vi "Untitled 3.vi"() -> ()   [LabVIEW 2017]
uses:
  8dd77c05-3ed4-427d-9456-dd24b11b0c44.vi
panel:
  out "<JSON>":string
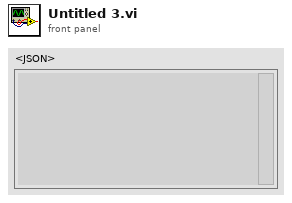
[diagram p1: front panel]
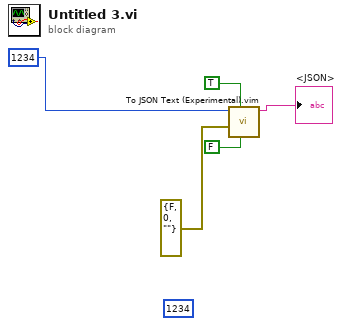
[diagram p0: block diagram]
diagram:
  (unwired) 1234
  n1 = call "To JSON Text (Experimental).vim"("Pretty Print?"=FALSE, "enable LabVIEW extensions? (T)"=TRUE, "error in (no error)"=errorcluster {"status"=FALSE, "code"=0, "source"=""}, "Anything"=1234) -> ("<JSON>"=→"<JSON>":string)  [unwired: 6 in, 1 out]
